vi "Gyro Turn.vi"(1 "setpoint":dbl format="%.2f") -> (6 "Left Motor":dbl format="%.2f", 9 "Right Motor":dbl format="%.2f")   [LabVIEW 2017]
uses:
  Drive Published Globals.vi
  <vilib>/addons/control/pid/pid.llb/PID (DBL).vi
  <vilib>/addons/control/pid/NI_PID_pid.lvlib
panel:
  in  "PID gains":T1={"proportional gain (Kc)"=1.0, "integral time (Ti, min)"=0.01, "derivative time (Td, min)"=0.0}
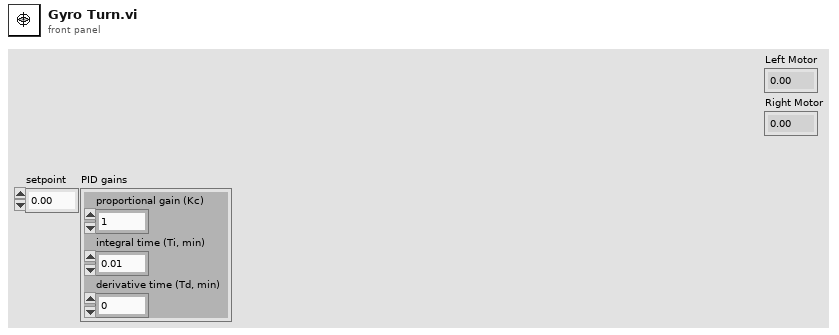
[diagram p1: front panel]
types:
  T1 = cluster{"proportional gain (Kc)":dbl, "integral time (Ti, min)":dbl, "derivative time (Td, min)":dbl}
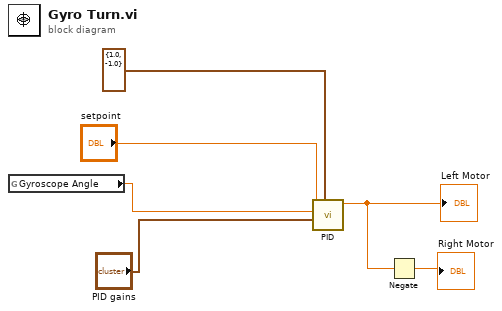
[diagram p0: block diagram]
diagram:
  n1 = global read "Drive Published Globals.vi" "Gyroscope Angle"() -> (w5:dbl)
  n2 = call-poly <vilib>:"PID.vi"("output range"=cluster{"output high":dbl, "output low":dbl} {"output high"=1.0, "output low"=-1.0}, "PID gains"="PID gains", "process variable"=w5, "setpoint"="setpoint") -> ("output"=w2:dbl)  [unwired: 6 in, 1 out]
  "Left Motor" <- w2
  n3 = Negate(x=w2) -> (-x=→"Right Motor":dbl)
